vi "Configured Acquisition Trigger (Host)_20230119.vi"() -> ()   [LabVIEW 2021]
doc: "Use this VI as a template to design an application that acquires data using advanced triggering logic from the NI PXIe-5170R/5171R."
uses:
  Device Session/Device Session.lvclass
  <vilib>/rvi/interface/nirviOpenFPGA/nirviOpenFPGA.xnode
  <vilib>/rvi/interface/nirviCloseFPGA/nirviCloseFPGA.xnode
  Enums/Channel Numbers.ctl
  <vilib>/FPGAPlugInAG/Dynamic/niLvFpga_Close_Dynamic.vi
  FPGA Bitfiles/Multirecord Acquisition FPGA_20221228a_4.lvbitx
  <vilib>/FPGAPlugInAG/PXIe-5172 (8CH - 410T)/niLvFpga_Open_PXIe-5172 (8CH - 410T).vi
  <vilib>/rvi/interface/common/dynamic/niFpgaDynamicAddResources.vi
panel:
  out "Host Loop Count":i32
  out "Waveform Graph 1":T1(graph)
  out "TrigCfg Array":T2(array[cluster])
  out "TrigCount":u32[](array[numeric])
  in  "ResetTrig":bool=TRUE
  in  "Sliding Window Trigger":cluster{"Range":dbl, "StartCenter":dbl}[](array[cluster])=[{"Range"=2.01, "StartCenter"=0.0}, {"Range"=0.01, "StartCenter"=0.0}, {"Range"=5.0, "StartCenter"=0.0}, {"Range"=5.0, "StartCenter"=0.0}, {"Range"=5.0, "StartCenter"=0.0}, {"Range"=5.0, "StartCenter"=0.0}, {"Range"=5.0, "StartCenter"=0.0}, {"Range"=5.0, "StartCenter"=0.0}]
  out "actual sample rate":dbl format="%#_6p"
  in  "onboard sample clock rate":dbl(ring)=200000000.0 items=["250 MHz"=250000000.0, "200 MHz"=200000000.0, "150 MHz"=150000000.0]
  in  "impedance":enum8{"Default", "1 mega ohm", "50 ohm"}(ring)
  in  "vertical offset (V)":dbl format="%.2p"
  out "Waveform Graph 0":T1(graph)
  in  "mode":T3(ring)
  in  "decimation factor":u16=1
  in  "coupling":enum8{"Default", "DC", "AC"}(ring)
  in  "bandwidth":T4(ring)
  in  "pretrigger samples":u64=500
  in  "number of samples":u64=1000
  in  "RIO Device":tag="PXI2Slot3"
  in  "channel(s)":string="0,1,2,3,4,5,6,7"
  in  "vertical range (Vpp)":dbl=1.0 format="%.2p"
  out "error out":errorcluster
  in  "stop":bool
  # "RIO Device"
  # "Vertical Settings"
  # "Trigger Settings"
  # "Acquisition Settings"
  # "DSP"
  # "Clocking"
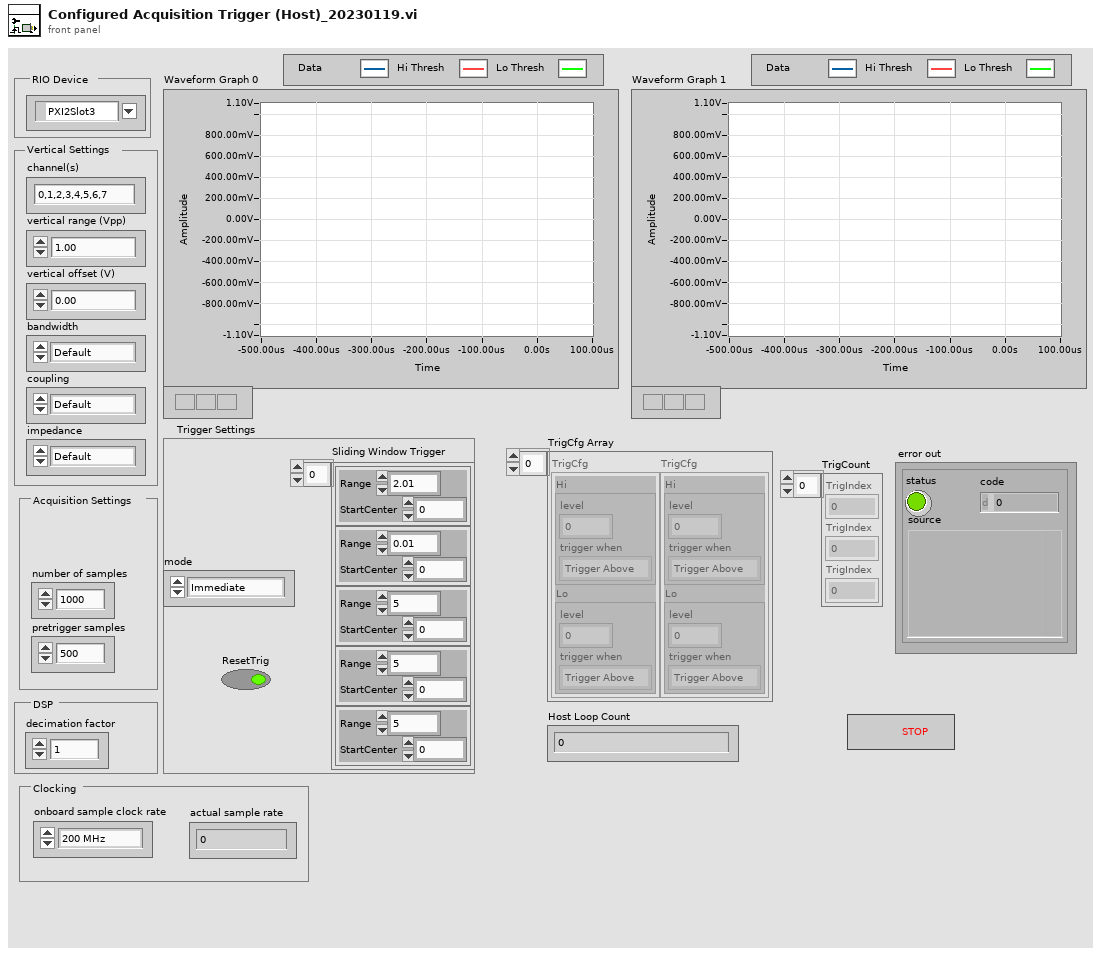
[diagram p1: front panel]
types:
  T1 = cluster{"relativeX":dbl, "sample rate":dbl, "data in":dbl[]}[]
  T2 = cluster{"Hi":cluster{"level":fxp<+/-,18,5>, "trigger when":enum8{"Trigger Above", "Trigger Below"}}, "Lo":cluster{"level":fxp<+/-,18,5>, "trigger when":enum8{"Trigger Above", "Trigger Below"}}}[]
  T3 = enum16{"Immediate", "A", "B", "OR", "AND", "A THEN B", "B THEN A", "High Resolution"}
  T4 = enum8{"Default", "Full Bandwidth", "Anti-alias Filter", "80 MHz FIR Filter", "40 MHz FIR Filter", "20 MHz FIR Filter"}
  T5 = typedef "Channel Numbers.ctl" = enum16{"0", "1", "2", "3", "4", "5", "6", "7"}
  T6 = typedef "niInstr Multirecord Acquisition v1 Host.lvclass/Scaling Coefficient.ctl" = cluster{"gain":dbl, "offset":dbl}
  T7 = typedef "ChannelWindowClust.ctl" = cluster{"HalfRange":fxp<+/-,18,5>, "StartCenter":fxp<+/-,18,5>}
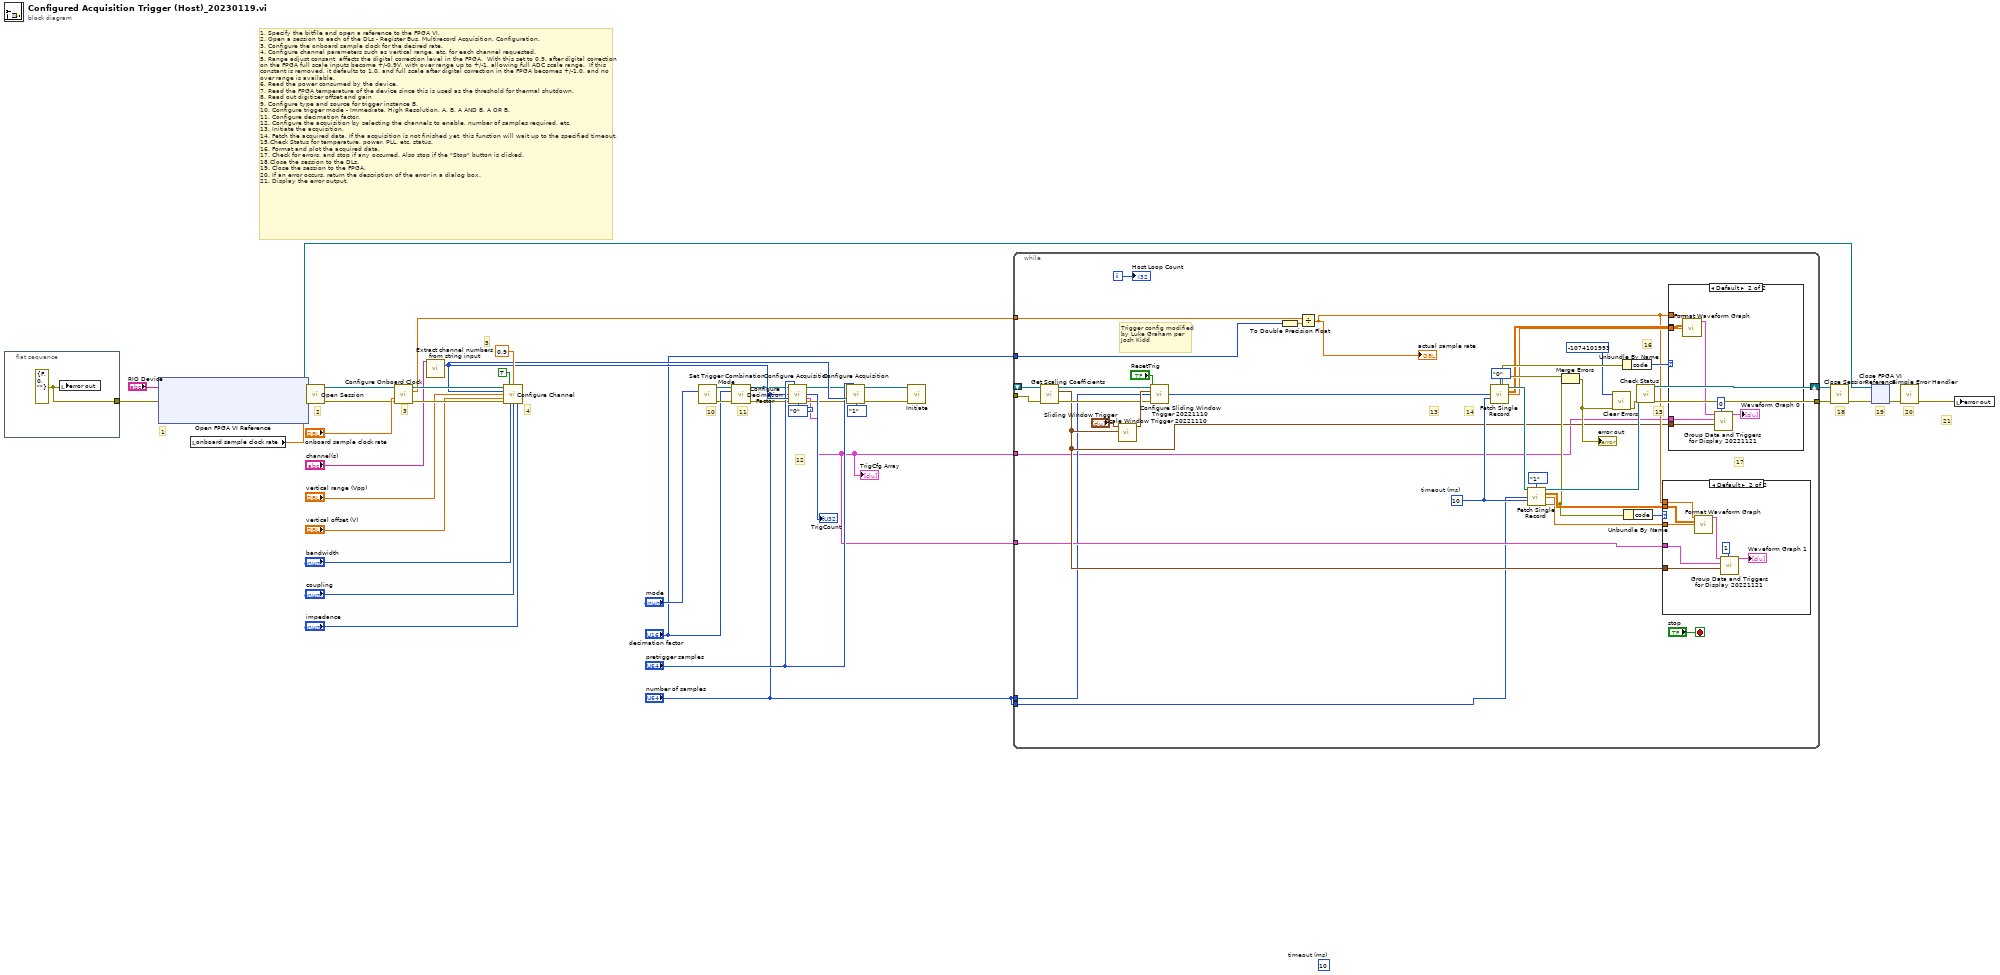
[diagram p0: block diagram]
diagram:
  (unwired) 10  # timeout (ms)
  # "11"
  # "10"
  # "12"
  # "4"
  # "5"
  # "3"
  # "21"
  # "20"
  # "19"
  # "18"
  # "1. Specify the bitfile and open a reference to the FPGA VI.\n2. Open a session to each of the DLs - Register Bus, Multirecord Acquisition, Configuration.\n3. Configure the onboard sample clock for the desired rate.\n4. Configure channel parameters such as vertical range, etc. for each channel requested.\n5. Range adjust consant  affects the digital correction level in the FPGA.  With this set to 0.9, after digital correction\non the FPGA full scale inputs become +/-0.9V, with over range up to +/-1, allowing full ADC scale range.  If this \nconstant is removed, it defaults to 1.0, and full scale after digital correction in the FPGA becomes +/-1.0, and no\nover range is available.  \n6. Read the power consumed by the device.\n7. Read the FPGA temperature of the device since this is used as the threshold for thermal shutdown.\n8. Read out digitizer offset and gain\n9. Configure type and source for trigger instance B.\n10. Configure trigger mode - Immediate, High Resolution, A, B, A AND B, A OR B.\n11. Configure decimation factor.\n12. Configure the acquisition by selecting the channels to enable, number of samples required, etc.\n13. Initiate the acquisition.\n14. Fetch the acquired data. If the acquisition is not finished yet, this function will wait up to the specified timeout.\n15.Check Status for temperature, power, PLL, etc. status. \n16. Format and plot the acquired data.\n17. Check for errors, and stop if any occurred. Also stop if the \"Stop\" button is clicked.\n18.Close the session to the DLs.\n19. Close the session to the FPGA.\n20. If an error occurs, return the description of the error in a dialog box.\n21. Display the error output."
  # "2"
  # "1"
  n1 = flat-sequence {
    tunnel: [w43] -> w34
    frame #0 {
      w43 = errorcluster {"status"=FALSE, "code"=0, "source"=""} ("error constant")
      n2 = local write "error out"(w43) -> ()
    }
  }
  n3 = xnode "Open FPGA VI Reference"("error in"=w34, "resource name"="RIO Device") -> ("FPGA VI Reference Out"=w38:refnum<k20>, "error out"=w33:errorcluster)
  n4 = local read "onboard sample clock rate"() -> (w36:dbl)
  n5 = call "Open Session.vi"("FPGA VI Ref"=w38, "adc clock rate (Hz)"=w36, "error in"=w33) -> ("device session out"=w23:refnum<class "Device Session.lvclass">, "error out"=w22:errorcluster)  [unwired: 11 in]
  n6 = call "Configure Onboard Clock.vi"("device session in"=w23, "adc clock rate (Hz)"="onboard sample clock rate", "error in"=w22) -> ("device session out"=w32:refnum<class "Device Session.lvclass">, "actual adc clock rate (Hz)"=w18:dbl, "error out"=w27:errorcluster)  [unwired: 9 in, 1 out]
  n7 = call "Extract channel numbers from string input.vi"("channel input"="channel(s)") -> ("array of chans"=w19:u32[])  [unwired: 13 in, 1 out]
  n8 = call "Configure Channel.vi"("device session in"=w32, "enable channel (T)"=TRUE ("enable channel"), "range adjust"=0.9, "channels"=w19, "vertical range (Vpp)"="vertical range (Vpp)", "vertical offset (V)"="vertical offset (V)", "error in"=w27, "bandwidth"="bandwidth", "coupling"="coupling", "impedance"="impedance") -> ()  [unwired: 4 in, 2 out]
  n9 = call "Set Trigger Combination Mode.vi"("mode"="mode") -> ("device session out"=w6:refnum<class "Device Session.lvclass">, "error out"=w7:errorcluster)  [unwired: 13 in]
  n10 = call "Configure Decimation Factor.vi"("device session in"=w6, "decimation factor"="decimation factor", "error in"=w7) -> ("device session out"=w9:refnum<class "Device Session.lvclass">, "error out"=w8:errorcluster)  [unwired: 11 in]
  n11 = call "Configure Acquisition.vi"("device session in"=w9, "pretrigger samples"="pretrigger samples", "number of samples"="number of samples", "channels to store"=w19, "error in"=w8, "Chan#"=Channel_Numbers."0") -> ("device session out"=w10:refnum<class "Device Session.lvclass">, "TrigCount"=→"TrigCount":u32[], "TrigCfg Array"=w3:T2, "error out"=w13:errorcluster)  [unwired: 5 in, 1 out]
  "TrigCfg Array" <- w3
  n12 = call "Configure Acquisition.vi"("device session in"=w10, "pretrigger samples"="pretrigger samples", "channels to store"=w19, "error in"=w13, "Chan#"=Channel_Numbers."1") -> ("device session out"=w11:refnum<class "Device Session.lvclass">, "number of samples"=w17:u64, "error out"=w12:errorcluster)  [unwired: 5 in, 3 out]
  n13 = call "Initiate.vi"("device session in"=w11, "error in"=w12) -> ()  [unwired: 12 in, 2 out]
  n14 = while {
    shift-right: [w77] -> w41
    shift-left: _ -> [w51]
    tunnel: [w75] -> w42
    tunnel: w18 -> [w61]
    tunnel: _ -> [w53]
    tunnel: w3 -> [w48]
    tunnel: w3 -> [w45]
    tunnel: "decimation factor" -> [w47]
    tunnel: "number of samples" -> [w46]
    tunnel: "number of samples" -> [w44]
    i -> [w56]
    stop <- "stop" stop-if-true
    w71 = 10  # timeout (ms)
    # "Trigger config modified by Luke Graham per Josh Kidd"
    # "15"
    # "17"
    # "16"
    # "14"
    # "13"
    n15 = call "Get Scaling Coefficients.vi"("device session in"=w51, "error in"=w53) -> ("device session out"=w50:refnum<class "Device Session.lvclass">, "scaling coefficients"=w49:T6[], "error out"=w52:errorcluster)  [unwired: 11 in]
    n16 = call "Scale Window Trigger 20221110.vi"("scaling coefficients"=w49, "Sliding Window Trigger"="Sliding Window Trigger") -> ("Sliding Window Trigger (FXP)"=w54:T7[])  [unwired: 9 in]
    n17 = call "Configure Sliding Window Trigger 20221110.vi"("device session in"=w50, "Sliding Window Triggers (FXP)"=w54, "ResetTrig"="ResetTrig", "error in"=w52) -> ()  [unwired: 10 in, 2 out]
    n18 = To Double Precision Float(number=w47) -> (double precision float=w78:dbl)
    n19 = Divide(x=w61, y=w78) -> (x/y=w57:dbl)
    "actual sample rate" <- w57
    n20 = call "Fetch Single Record.vi"("number of samples"=w46, "timeout (ms)"=w71, "Chan#"=Channel_Numbers."0") -> ("device session out"=w73:refnum<class "Device Session.lvclass">, "data"=w60:dbl[][], "relativeX (samples)"=w59:dbl, "error out"=w67:errorcluster)  [unwired: 8 in, 1 out]
    n21 = call "Fetch Single Record.vi"("device session in"=w73, "number of samples"=w44, "timeout (ms)"=w71, "Chan#"=Channel_Numbers."1") -> ("device session out"=w72:refnum<class "Device Session.lvclass">, "data"=w70:dbl[][], "relativeX (samples)"=w58:dbl, "error out"=w62:errorcluster)  [unwired: 7 in, 1 out]
    n22 = Merge Errors(w67, w62) -> (w66:errorcluster)
    "error out" <- w66
    n23 = call <vilib>:"Clear Errors.vi"("error in (no error)"=w66, "specific error code to clear (0: all)"=-1074101993) -> ("error out"=w65:errorcluster)  [unwired: 4 in, 1 out]
    n24 = Unbundle By Name(w67) -> ("code"=w68:i32)
    n25 = Unbundle By Name(w62) -> ("code"=w63:i32)
    n26 = call "Check Status.vi"("device session in"=w72, "error in"=w65) -> ("device session out"=w77:refnum<class "Device Session.lvclass">, "error out"=w75:errorcluster)  [unwired: 12 in]
    n27 = case shown="Default" w63 {
      tunnel: w70 -> [_ w86]
      tunnel: w48 -> [_ w87]
      tunnel: w49 -> [_ w83]
      tunnel: w58 -> [_ w81]
      tunnel: w57 -> [_ w80]
      frame -1074101998, -1074101995, -1074101993 {
      }
      frame Default {
        n28 = call "Format Waveform Graph.vi"("sample rate (Hz)"=w80, "data in"=w86, "relativeX (samples)"=w81) -> ("waveform out"=w85:T1)  [unwired: 12 in]
        n29 = call "Group Data and Triggers for Display 20221121.vi"("Chan"=1, "scaling coefficients"=w83, "TrigCfg"=w87, "Data waveform"=w85) -> ("Data for Display"=→"Waveform Graph 1":T1)  [unwired: 7 in]
      }
    }
    n30 = case shown="Default" w68 {
      tunnel: w45 -> [_ w93]
      tunnel: w49 -> [_ w94]
      tunnel: w57 -> [_ w92]
      tunnel: w60 -> [_ w91]
      tunnel: w59 -> [_ w90]
      frame -1074101998, -1074101995, -1074101993 {
      }
      frame Default {
        n31 = call "Format Waveform Graph.vi"("sample rate (Hz)"=w92, "data in"=w91, "relativeX (samples)"=w90) -> ("waveform out"=w89:T1)  [unwired: 12 in]
        n32 = call "Group Data and Triggers for Display 20221121.vi"("Chan"=0, "scaling coefficients"=w94, "TrigCfg"=w93, "Data waveform"=w89) -> ("Data for Display"=→"Waveform Graph 0":T1)  [unwired: 7 in]
      }
    }
    "Host Loop Count" <- w56
  }
  n33 = call "Close Session.vi"("device session in"=w41, "error in"=w42) -> ("error out"=w39:errorcluster)  [unwired: 13 in]
  n34 = xnode "Close FPGA VI Reference"("FPGA VI Reference In"=w38, "error in"=w39) -> ("error out"=w37:errorcluster)
  n35 = call <vilib>:"Simple Error Handler.vi"("error in (no error)"=w37) -> ("error out"=w35:errorcluster)  [unwired: 4 in, 4 out]
  n36 = local write "error out"(w35) -> ()
